vi "Biot-Savart induced velocity.vi"(1 "E":sgl[](array[numeric]), 2 "P1":sgl[](array[numeric]), 3 "P0":sgl[](array[numeric]), 4 "P":sgl[](array[numeric])) -> (0 "U / G'":sgl[](array[numeric]))   [LabVIEW 2017]
doc: "P is the point of interest\nP0 is the start-point of the filament edge\nP1 is the end-point of the filament edge\nE is the filament edge vector (P1 - P0)\n\nOutput = U_induced / Gamma'"
panel:
  # "PN 22/10/17"
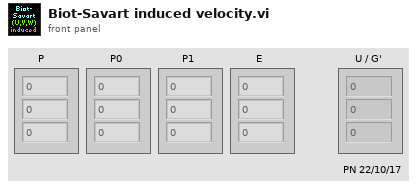
[diagram p1: front panel]
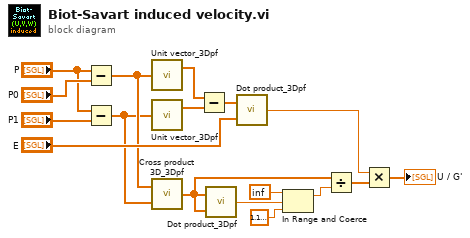
[diagram p0: block diagram]
diagram:
  n1 = Subtract(x="P", y="P0") -> (x-y=w10:sgl[])
  n2 = Subtract(x="P", y="P1") -> (x-y=w9:sgl[])
  n3 = call "Unit vector_3Dpf.vi"("Vector"=w10) -> ("Unit vector"=w14:sgl[])  [unwired: 1 out]
  n4 = call "Unit vector_3Dpf.vi"("Vector"=w9) -> ("Unit vector"=w13:sgl[])  [unwired: 1 out]
  n5 = call "Cross product 3D_3Dpf.vi"("B"=w9, "A"=w10) -> ("A x B"=w8:sgl[])
  n6 = Subtract(x=w14, y=w13) -> (x-y=w11:sgl[])
  n7 = call "Dot product_3Dpf.vi"("B"=w8, "A"=w8) -> ("A . B"=w2:sgl)
  n8 = call "Dot product_3Dpf.vi"("B"="E", "A"=w11) -> ("A . B"=w7:sgl)
  n9 = In Range and Coerce(upper limit=sgl inf, x=w2, lower limit=sgl 1.1920929e-07) -> (coerced(x)=w1:sgl)  [unwired: 1 out]
  n10 = Divide(x=w8, y=w1) -> (x/y=w6:sgl[])
  n11 = Multiply(x=w7, y=w6) -> (x*y=→"U / G'":sgl[])
